vi "Zero Phase Lowpass Filter (multiple).vi"(8 "error in (no error)":errorcluster, 10 "cutoff period":dbl, 11 "XY-data":cluster{"X-array":dbl[], "Y-array":dbl[]}[](array[cluster])) -> (0 "error out":errorcluster, 3 "XY-data out":cluster{"X-array":dbl[], "Y-array":dbl[]}[](array[cluster]) {"Y-array" format="%.2p"; "X-array" format="%.2p"})   [LabVIEW 2016, in "xy_utilities.lvlib"]
doc: "Apply a Zero Phase Lowpass Filter to <b>XY-Data<b/>'s Y-Array.\n\n<b>cutoff period</b> is equivalent to 1/cutoff frequency and is in the units of the X-Array. The cutoff frequency is restricted between 0 and Fs/4.\n\nWire data to the data input to determine the polymorphic instance to use or manually select the instance."
uses:
  xy_utilities.lvlib
  Private/Get X Array dx.vi
  <vilib>/Utility/error.llb/Error Cluster From Error Code.vi
  <vilib>/Analysis/3filter.llb/Zero Phase Filter.vi
  <vilib>/Analysis/3filter.llb/Zero Phase Filter (DBL).vi
  <vilib>/Analysis/3filter.llb/FIR Windowed Coefficients.vi
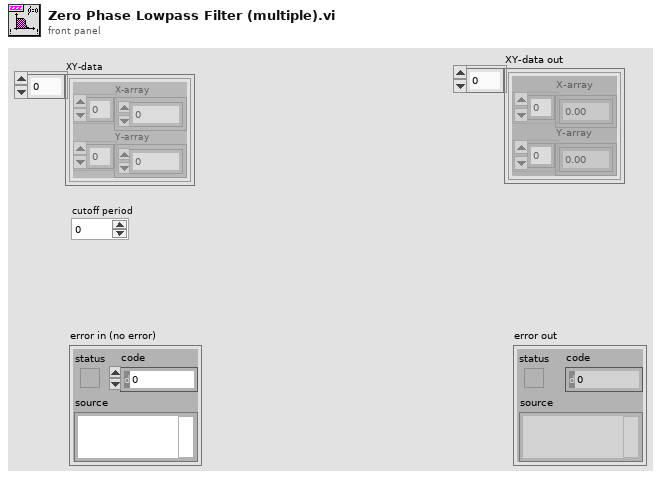
[diagram p1: front panel]
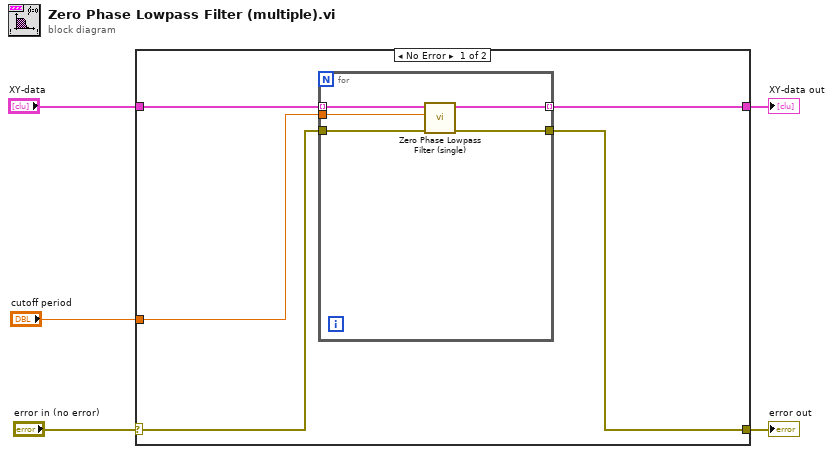
[diagram p0: block diagram]
diagram:
  n1 = case shown="No Error" "error in (no error)" {
    selector: "error in (no error)" -> [w7 w17]
    tunnel: [w6 w17] -> w4
    tunnel: "XY-data" -> [w10 w16]
    tunnel: [w9 w16] -> w2
    tunnel: "cutoff period" -> [w8 _]
    frame No Error {
      n2 = for {
        tunnel: w10 -> [w15] mode=indexing
        tunnel: [w14] -> w9 mode=indexing
        tunnel: w8 -> [w13]
        tunnel: w7 -> [w12]
        tunnel: [w11] -> w6
        n3 = call "Zero Phase Lowpass Filter (single).vi"("error in (no error)"=w12, "cutoff period"=w13, "XY-data"=w15) -> ("error out"=w11:errorcluster, "XY-data out"=w14:cluster{"X-array":dbl[], "Y-array":dbl[]})  [unwired: 7 in]
      }
    }
    frame Error {
    }
  }
  "error out" <- w4
  "XY-data out" <- w2
